vi "loop_opamp.vi"() -> ()   [LabVIEW 2020]
uses:
  2edfc998-1a2a-4353-bd21-6350e2ff24f5.vi
  <vilib>/Analysis/baseanly.llb/Mean (DBL).vi
  <vilib>/Utility/file.llb/Write Delimited Spreadsheet (DBL).vi
  <vilib>/Analysis/NI_AALBase.lvlib
panel:
  out "# iteration":dbl
  in  "Save data?":bool=TRUE
  out "log path":string
  in  "file name":string="prova_opamp"
  in  "?":bool
  out "V_MPP":dbl
  out "I_MPP":dbl
  out "index max power":i32
  out "max power":dbl
  in  "Tab Control":enum32{"Page 1"}(tab)
  out "Power":dbl[](graph)
  out "IV-PV":cluster{dbl[], dbl[]}[](graph)
  out "power [mW]":dbl
  out "voltage [V]":dbl format="%0.2f"
  out "current [mA]":dbl
  in  "battery voltage [V]":dbl=2.8 format="%#_13g"
  in  "resistance [kohm]":dbl=0.098
  in  "# points":i32=3
  out "V_opamp":dbl
  out "error out":errorcluster
  in  "V_stop":dbl=0.15
  in  "V_step":dbl=0.001
  in  "V_start":dbl
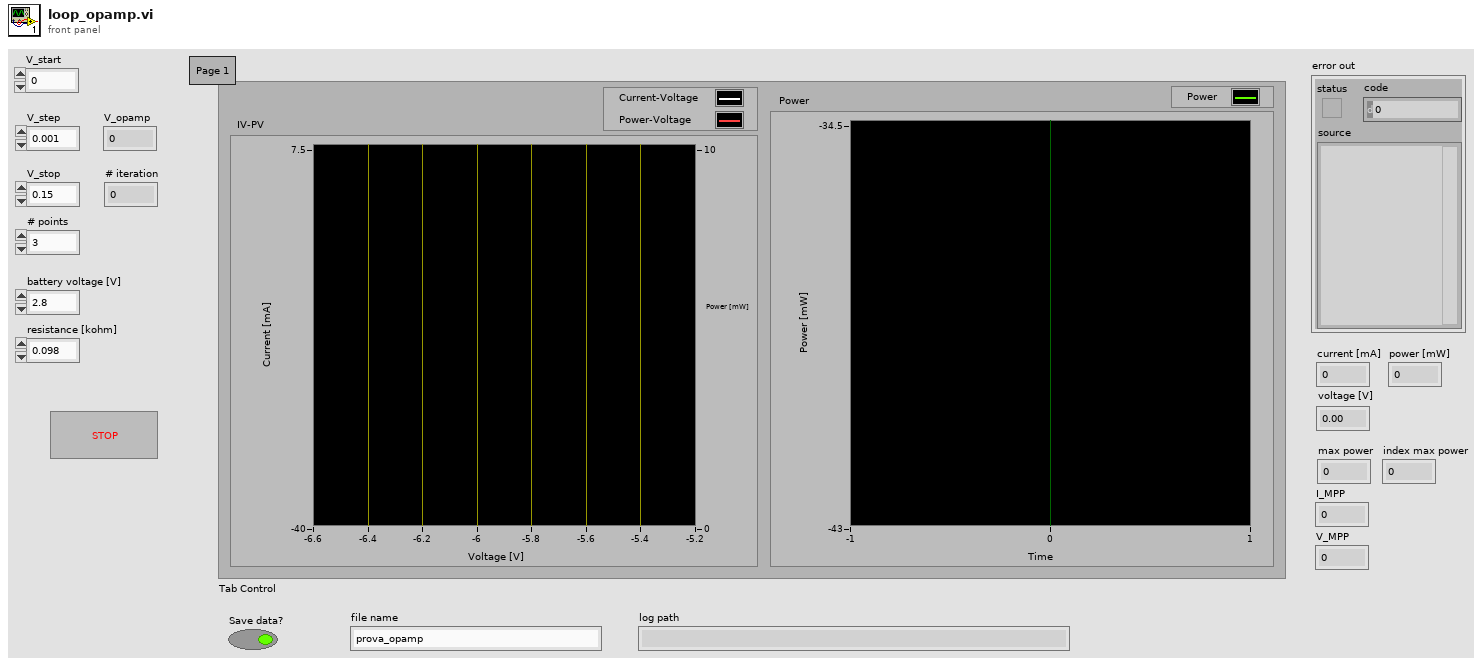
[diagram p1: front panel]
types:
  T1 = enum16{"open", "replace", "create", "open or create", "replace or create", "replace or create with confirmation"}
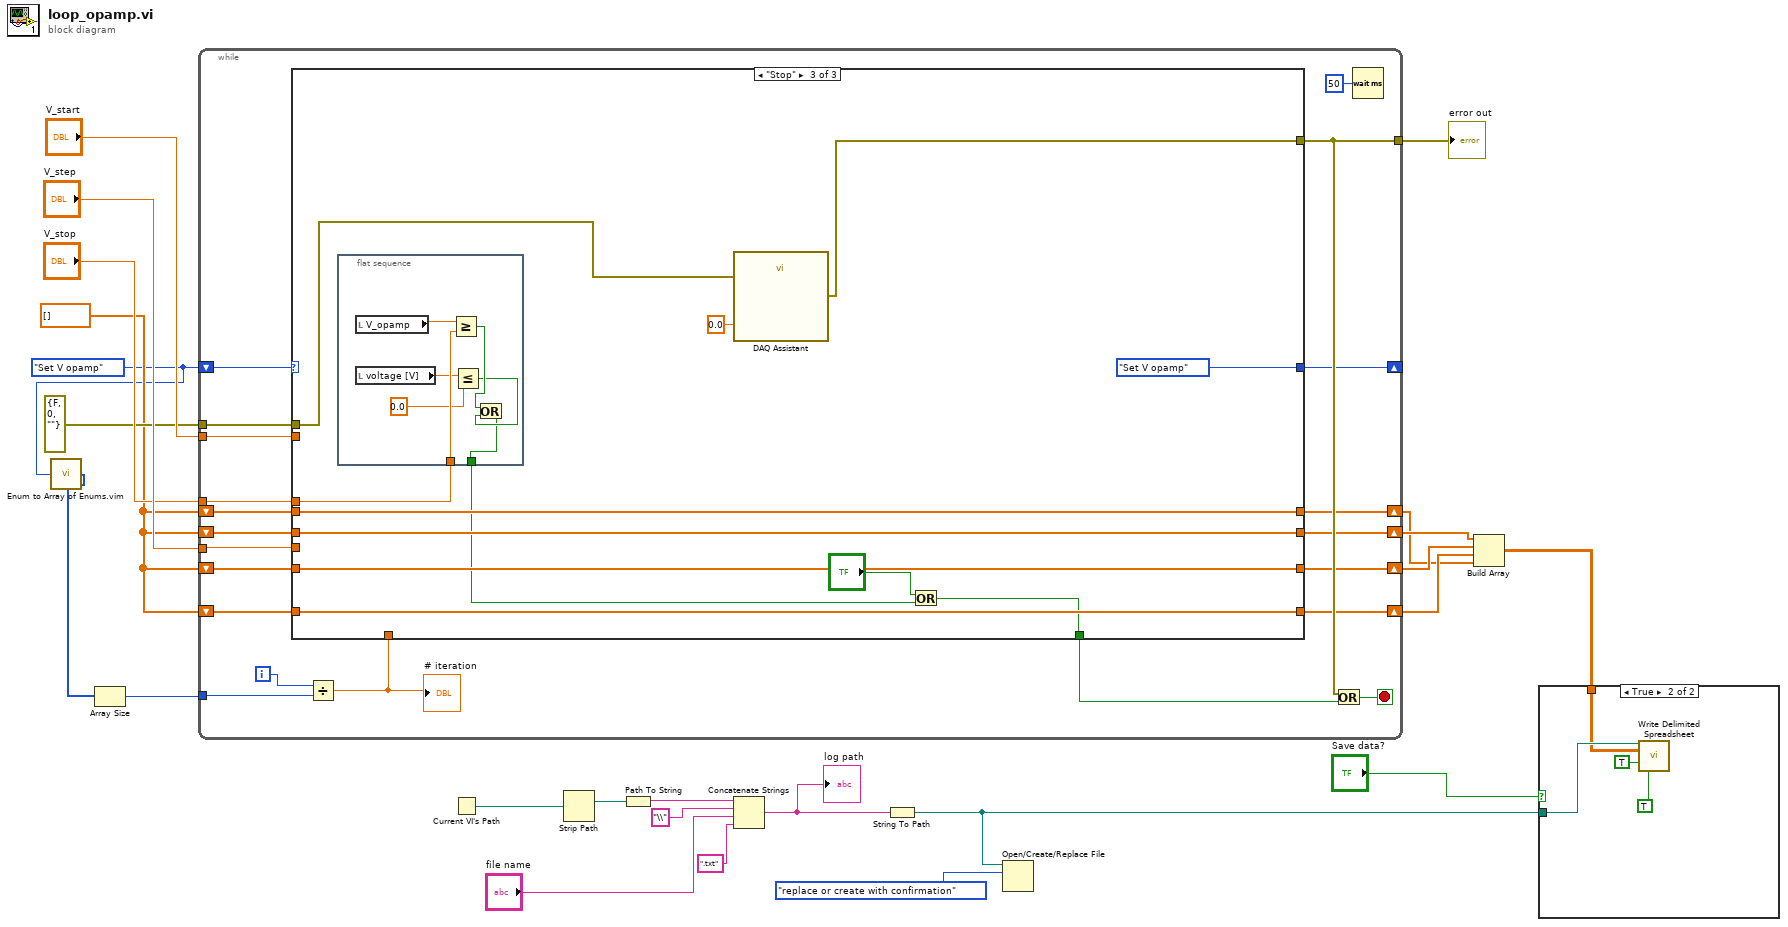
[diagram p0: block diagram]
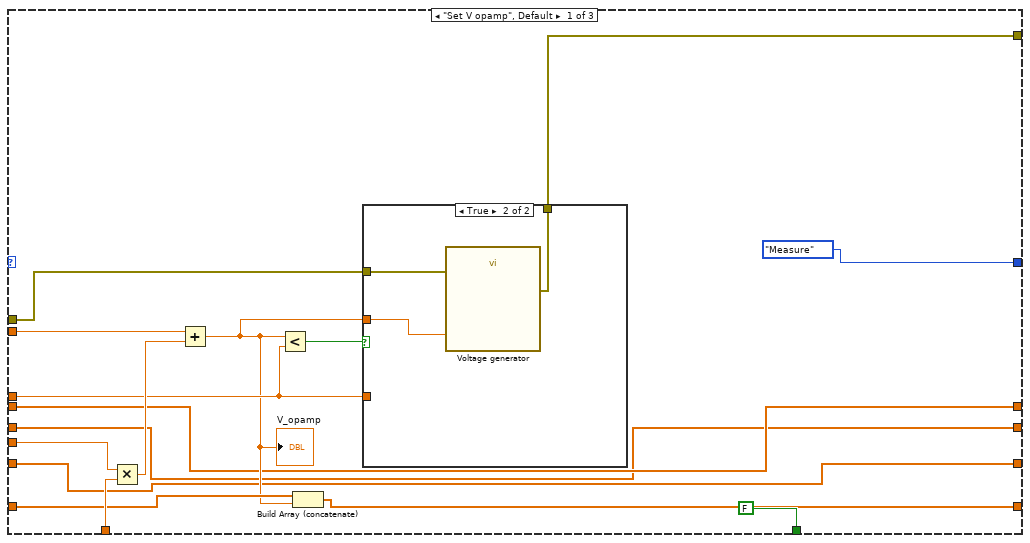
[diagram p3: hidden frame]
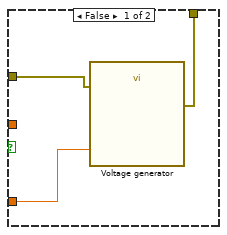
[diagram p4: hidden frame]
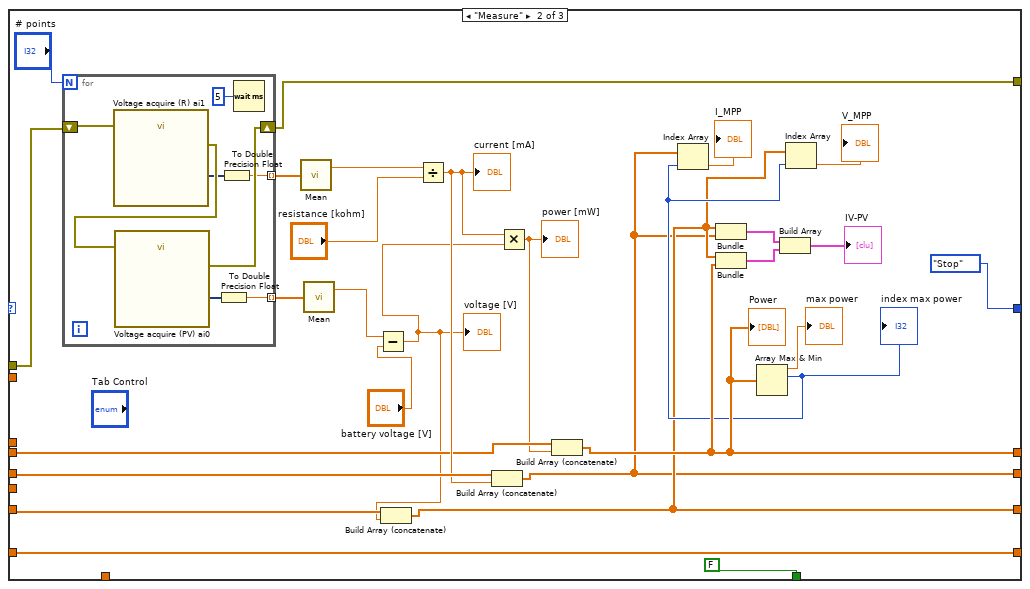
[diagram p5: hidden frame]
diagram:
  w19 = dbl[] []
  w3 = enum16{"Set V opamp", "Measure", "Stop"}."Set V opamp"
  n1 = call "Enum to Array of Enums.vim"("enum"=w3) -> ("array of enums"=w2:enum16{"Set V opamp", "Measure", "Stop"}[])
  n2 = Array Size(array=w2) -> (size(s)=w1:i32)
  n3 = while {
    tunnel: "V_start" -> [w43]
    tunnel: "V_step" -> [w41]
    tunnel: "V_stop" -> [w40]
    tunnel: errorcluster {"status"=FALSE, "code"=0, "source"=""} ("error in") -> [w39]
    tunnel: [w37] -> w20
    shift-right: [w34] -> w6
    shift-left: w19 -> [w35]
    shift-right: [w32] -> w7
    shift-left: w19 -> [w33]
    shift-right: [w30] -> w8
    shift-left: w19 -> [w31]
    shift-right: [w28] -> w5
    shift-left: w19 -> [w29]
    shift-right: [w27] -> _
    shift-left: w3 -> [w45]
    tunnel: w1 -> [w26]
    i -> [w42]
    stop <- w38 stop-if-true
    n4 = Divide(x=w42, y=w26) -> (x/y=w25:dbl)
    "# iteration" <- w25
    n5 = case shown="\"Stop\"" w45 {
      tunnel: w43 -> [w61 _ _]
      tunnel: w25 -> [w60 _ _]
      tunnel: w41 -> [w59 _ _]
      tunnel: w40 -> [w54 _ w111]
      tunnel: w39 -> [w56 w94 w106]
      tunnel: [w55 w93 w105] -> w37
      tunnel: [FALSE FALSE w108] -> w36
      tunnel: w35 -> [w52 w89 w112]
      tunnel: [w50 w89 w112] -> w34
      tunnel: [w47 w73 w113] -> w32
      tunnel: w33 -> [w47 w88 w113]
      tunnel: w31 -> [w48 w86 w114]
      tunnel: [w48 w72 w114] -> w30
      tunnel: w29 -> [w49 w84 w115]
      tunnel: [w49 w79 w115] -> w28
      tunnel: [enum16{"Set V opamp", "Measure", "Stop"}."Measure" enum16{"Set V opamp", "Measure", "Stop"}."Stop" enum16{"Set V opamp", "Measure", "Stop"}."Set V opamp"] -> w27
      frame "Set V opamp", Default {
        n6 = Multiply(x=w59, y=w60) -> (x*y=w58:dbl)
        n7 = Add(x=w61, y=w58) -> (x+y=w51:dbl)
        "V_opamp" <- w51
        n8 = Less?(x=w51, y=w54) -> (x < y?=w57:bool)
        n9 = Build Array (concatenate)(w52, w51) -> (w50:dbl[])
        n10 = case shown="True" w57 {
          tunnel: w51 -> [_ w67]
          tunnel: w56 -> [w63 w66]
          tunnel: [w62 w65] -> w55
          tunnel: w54 -> [w64 _]
          frame False {
            n11 = call "Voltage generator"("data"=w64, "error in"=w63) -> ("error out"=w62:errorcluster)  [unwired: 16 in, 1 out]
          }
          frame True {
            n12 = call "Voltage generator"("data"=w67, "error in"=w66) -> ("error out"=w65:errorcluster)  [unwired: 16 in, 1 out]
          }
        }
      }
      frame "Measure" {
        n13 = for {
          N: "# points" -> [_]
          shift-right: [w101] -> w93
          shift-left: w94 -> [w103]
          tunnel: [w98] -> w92 mode=indexing
          tunnel: [w97] -> w91 mode=indexing
          n14 = call "Voltage acquire (R) ai1"("error in"=w103) -> ("data"=w99:dynamicdata, "error out"=w102:errorcluster)  [unwired: 16 in, 1 out]
          n15 = call "Voltage acquire (PV) ai0"("error in"=w102) -> ("data"=w100:dynamicdata, "error out"=w101:errorcluster)  [unwired: 16 in, 1 out]
          n16 = To Double Precision Float(number=w100) -> (double precision float=w97:dbl)
          n17 = To Double Precision Float(number=w99) -> (double precision float=w98:dbl)
          n18 = Wait (ms)(milliseconds to wait=u32 5) -> ()  [unwired: 1 out]
        }
        n19 = call-poly <vilib>:"Mean.vi"("X"=w92) -> ("mean"=w71:dbl)  [unwired: 1 out]
        n20 = call-poly <vilib>:"Mean.vi"("X"=w91) -> ("mean"=w70:dbl)  [unwired: 1 out]
        n21 = Subtract(x=w70, y="battery voltage [V]") -> (x-y=w68:dbl)
        "voltage [V]" <- w68
        n22 = Build Array (concatenate)(w88, w68) -> (w73:dbl[])
        n23 = Divide(x=w71, y="resistance [kohm]") -> (x/y=w85:dbl)
        "current [mA]" <- w85
        n24 = Build Array (concatenate)(w86, w85) -> (w72:dbl[])
        n25 = Multiply(x=w85, y=w68) -> (x*y=w83:dbl)
        "power [mW]" <- w83
        n26 = Build Array (concatenate)(w84, w83) -> (w79:dbl[])
        "Power" <- w79
        n27 = Bundle(w73, w72) -> (w82:cluster{dbl[], dbl[]})  [unwired: 1 in]
        n28 = Bundle(w73, w79) -> (w81:cluster{dbl[], dbl[]})  [unwired: 1 in]
        n29 = Array Max & Min(array=w79) -> (max value=→"max power":dbl, max index (indices)=w76:i32)  [unwired: 2 out]
        "index max power" <- w76
        n30 = Index Array(array=w72, index=w76) -> (element=→"I_MPP":dbl)
        n31 = Build Array(w82, w81) -> (→"IV-PV":cluster{dbl[], dbl[]}[])
        n32 = Index Array(array=w73, index=w76) -> (element=→"V_MPP":dbl)
      }
      frame "Stop" {
        n33 = flat-sequence {
          tunnel: w111 -> [w121]
          tunnel: [w117] -> w109
          frame #0 {
            n34 = local read "V_opamp"() -> (w122:dbl)
            n35 = local read "voltage [V]"() -> (w120:dbl)
            n36 = Greater Or Equal?(x=w122, y=w121) -> (x >= y?=w119:bool)
            n37 = Less Or Equal?(x=w120, y=0.0) -> (x <= y?=w118:bool)
            n38 = Or(x=w119, y=w118) -> (x .or. y?=w117:bool)
          }
        }
        n39 = call "DAQ Assistant"("data"=0.0, "error in"=w106) -> ("error out"=w105:errorcluster)  [unwired: 16 in, 1 out]
        n40 = Or(x="?", y=w109) -> (x .or. y?=w108:bool)
      }
    }
    n41 = Or(x=w37, y=w36) -> (x .or. y?=w38:bool)
    n42 = Wait (ms)(milliseconds to wait=u32 50) -> ()  [unwired: 1 out]
  }
  "error out" <- w20
  n43 = Current VI's Path() -> (path=w18:path)
  n44 = Strip Path(path=w18) -> (stripped path=w17:path)  [unwired: 1 out]
  n45 = Path To String(path=w17) -> (string=w16:string)
  n46 = Concatenate Strings(w16, "\\" ("string"), "file name", ".txt" ("string")) -> (w12:string)
  "log path" <- w12
  n47 = String To Path(string=w12) -> (path=w9:path)
  n48 = Open/Create/Replace File(file path (use dialog)=w9, operation (0:open)=T1."replace or create with confirmation") -> ()  [unwired: 4 in, 3 out]
  n49 = Build Array(w8, w7, w6, w5) -> (w4:dbl[][])
  n50 = case shown="True" "Save data?" {
    tunnel: w9 -> [_ w126]
    tunnel: w4 -> [_ w125]
    frame False {
    }
    frame True {
      n51 = call-poly <vilib>:"Write Delimited Spreadsheet.vi"("file path (dialog if empty)"=w126, "2D data"=w125, "append to file? (new file:F)"=TRUE, "transpose? (no:F)"=TRUE) -> ()  [unwired: 10 in, 2 out]
    }
  }
